vi "IncrementArrayElement.vi"(10 "Index":i32, 11 "Histogram in":u16[](array[numeric])=[0, 0, 0, 0, 0, 0, 0, 0, 0, 0]) -> (3 "Histogram out":u16[](array[numeric]))   [LabVIEW 2012]
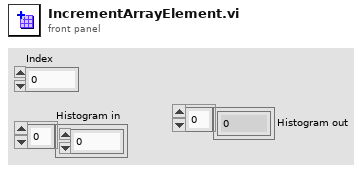
[diagram p1: front panel]
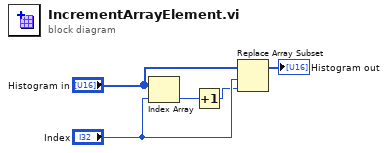
[diagram p0: block diagram]
diagram:
  n1 = Index Array(array="Histogram in", index="Index") -> (element=w4:u16)
  n2 = Increment(x=w4) -> (x+1=w3:u16)
  n3 = Replace Array Subset(array="Histogram in", new element=w3, index="Index") -> (→"Histogram out":u16[])
